vi "ueye open camera.vi"(8 "error in (no error)":errorcluster, 10 "Camera Settings":path, 11 "identifier":string) -> (0 "error out":errorcluster, 3 "Camera reference out":refnum<k24>)   [LabVIEW 2023, in "Vision.lvlib"]
uses:
  Vision.lvlib
  C:/Users/cfangmeier3/Desktop/nebraska-silicon-lab/pixel-gantry-control/Gantry/Shared Components/bin/uEyeDotNet.dll
  bin/uEyeDotNet.dll
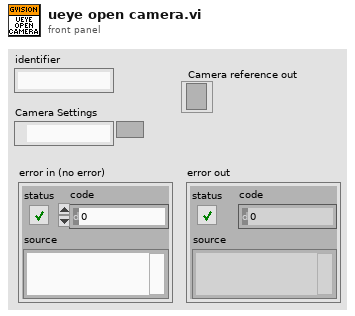
[diagram p1: front panel]
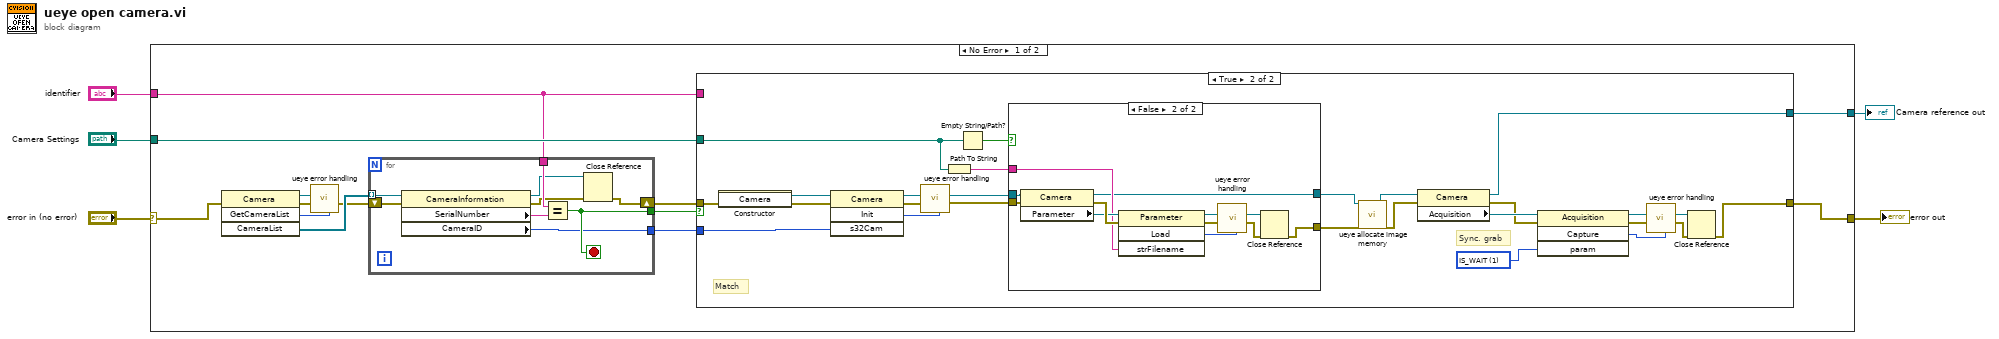
[diagram p0: block diagram]
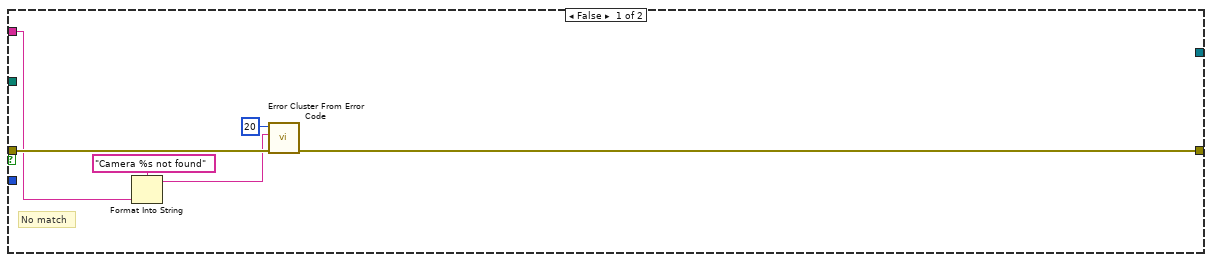
[diagram p2: hidden frame]
diagram:
  n1 = case shown="No Error" "error in (no error)" {
    selector: "error in (no error)" -> [w10 w71]
    tunnel: "Camera Settings" -> [w9 _]
    tunnel: "identifier" -> [w8 _]
    tunnel: [w7 w71] -> w2
    tunnel: [w6 _] -> w1
    frame No Error {
      n2 = invoke on="Methodenknoten" class="Camera" method="GetCameraList"(error in=w10) -> (reference out=w11:refnum<k24>, error out=w14:errorcluster, "GetCameraList"=w12:i32, "CameraList"=w18:refnum<k24>[])  [unwired: 3 in]
      n3 = call "ueye error handling.vi"("Error Code"=w12, "reference in"=w11, "Error In"=w14) -> ("Error Out"=w13:errorcluster)  [unwired: 8 in]
      n4 = for {
        tunnel: w18 -> [w70] mode=indexing
        tunnel: w8 -> [w69]
        tunnel: [w67] -> w17
        shift-right: [w63] -> w16
        shift-left: w13 -> [w66]
        tunnel: [w65] -> w15
        stop <- w67 stop-if-true
        n5 = property class="CameraInformation"(reference=w70, error in=w66) -> (reference out=w62:refnum<k24>, error out=w64:errorcluster, "SerialNumber"=w68:string, "CameraID"=w65:i64)
        n6 = Equal?(x=w69, y=w68) -> (x = y?=w67:bool)
        n7 = Close Reference(reference=w62, error in (no error)=w64) -> (error out=w63:errorcluster)
      }
      n8 = case shown="True" w17 {
        tunnel: w16 -> [w24 w48]
        tunnel: w15 -> [_ w46]
        tunnel: [w23 w28] -> w7
        tunnel: w8 -> [w20 _]
        tunnel: w9 -> [_ w26]
        tunnel: [_ w27] -> w6
        frame False {
          # "No match"
          n9 = Format Into String(format string="Camera %s not found" ("error message (\"\")"), w20) -> (resulting string=w19:string)  [unwired: 2 in, 1 out]
          n10 = call <vilib>:"Error Cluster From Error Code.vi"("error in (no error)"=w24, "error message (\"\")"=w19, "error code (0)"=20) -> ("error out"=w23:errorcluster)  [unwired: 6 in]
        }
        frame True {
          w42 = 1 items=["IS_DONT_WAIT", "IS_WAIT"] ("Wait")
          # "Sync. grab"
          # "Match"
          n11 = constructor class="Camera"(error in=w48) -> (reference out=w40:refnum<k24>, error out=w47:errorcluster)  [unwired: 2 in, 1 out]
          n12 = invoke class="Camera" method="Init"(reference=w40, error in=w47, "s32Cam"=w46) -> (reference out=w35:refnum<k24>, error out=w45:errorcluster, "Init"=w36:i32)  [unwired: 1 in, 1 out]
          n13 = call "ueye error handling.vi"("Error Code"=w36, "reference in"=w35, "Error In"=w45) -> ("Error Out"=w39:errorcluster)  [unwired: 8 in]
          n14 = Path To String(path=w26) -> (string=w41:string)
          n15 = Empty String/Path?(string/path=w26) -> (empty?=w25:bool)
          n16 = case shown="False" w25 {
            tunnel: w41 -> [_ w59]
            tunnel: w39 -> [w49 w58]
            tunnel: [w50 w57] -> w37
            tunnel: w35 -> [w50 w54]
            tunnel: [w49 w52] -> w32
            frame True {
            }
            frame False {
              n17 = property class="Camera"(reference=w54, error in=w58) -> (reference out=w57:refnum<k24>, error out=w61:errorcluster, "Parameter"=w60:refnum<k24>)
              n18 = invoke class="Parameter" method="Load"(reference=w60, error in=w61, "strFilename"=w59) -> (reference out=w51:refnum<k24>, error out=w55:errorcluster, "Load"=w56:i32)  [unwired: 1 in, 1 out]
              n19 = call "ueye error handling.vi"("Error Code"=w56, "reference in"=w51, "Error In"=w55) -> ("Error Out"=w53:errorcluster)  [unwired: 8 in]
              n20 = Close Reference(reference=w51, error in (no error)=w53) -> (error out=w52:errorcluster)
            }
          }
          n21 = call "ueye allocate image memory.vi"("Camera reference in"=w37, "Error In"=w32) -> ("Camera reference out"=w31:refnum<k24>, "Error Out"=w38:errorcluster)  [unwired: 12 in, 4 out]
          n22 = property class="Camera"(reference=w31, error in=w38) -> (reference out=w27:refnum<k24>, error out=w43:errorcluster, "Acquisition"=w44:refnum<k24>)
          n23 = invoke class="Acquisition" method="Capture"(reference=w44, error in=w43, "param"=w42) -> (reference out=w30:refnum<k24>, error out=w34:errorcluster, "Capture"=w33:i32)  [unwired: 1 in, 1 out]
          n24 = call "ueye error handling.vi"("Error Code"=w33, "reference in"=w30, "Error In"=w34) -> ("Error Out"=w29:errorcluster)  [unwired: 8 in]
          n25 = Close Reference(reference=w30, error in (no error)=w29) -> (error out=w28:errorcluster)
        }
      }
    }
    frame Error {
    }
  }
  "error out" <- w2
  "Camera reference out" <- w1
